vi "MD5 vs FileDateSize Check.vi"() -> ()   [LabVIEW 2016]
panel:
  out "x-y":u32
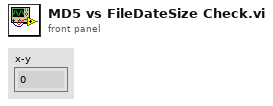
[diagram p1: front panel]
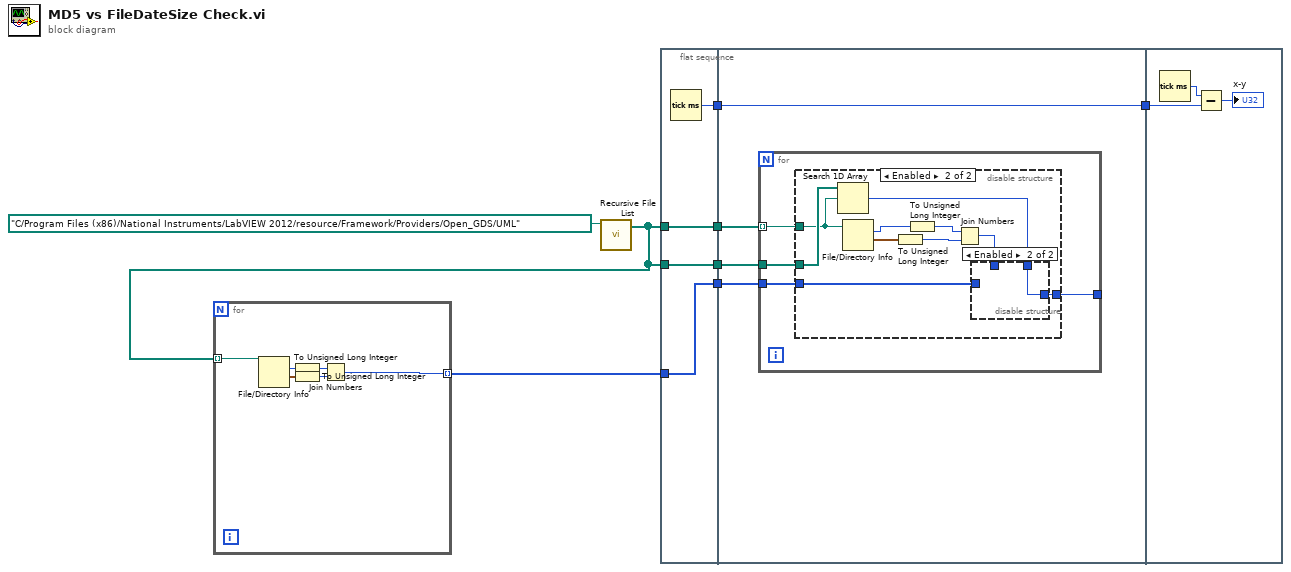
[diagram p0: block diagram]
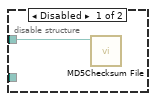
[diagram p2: hidden frame]
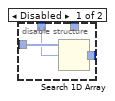
[diagram p3: hidden frame]
diagram:
  n1 = call <vilib>:"Recursive File List.vi"("Folder Path"=path "C:/Program Files (x86)/National Instruments/LabVIEW 2012/resource/Framework/Providers/Open_GDS/UML") -> ("All Files in Dir"=w2:path[])  [unwired: 6 in, 4 out]
  n2 = for {
    tunnel: w2 -> [w14] mode=indexing
    tunnel: [w13] -> w4 mode=indexing
    n3 = File/Directory Info(path=w14) -> (size=w11:i64, last mod=w12:timestamp)  [unwired: 1 in, 5 out]
    n4 = To Unsigned Long Integer(number=w11) -> (unsigned 32bit integer=w10:u32)
    n5 = To Unsigned Long Integer(number=w12) -> (unsigned 32bit integer=w9:u32)
    n6 = Join Numbers(hi=w10, lo=w9) -> ((hi.lo)=w13:u64)
  }
  n7 = flat-sequence {
    tunnel: [w18] -> w8
    tunnel: w2 -> [w17]
    tunnel: [w17] -> w5
    tunnel: w4 -> [w16]
    tunnel: [w16] -> w3
    tunnel: w2 -> [w15]
    tunnel: [w15] -> w1
    tunnel: w8 -> [w22]
    tunnel: [w22] -> w7
    tunnel: w5 -> [w21]
    tunnel: w3 -> [w20]
    tunnel: w1 -> [w19]
    tunnel: w7 -> [w43]
    frame #0 {
      n8 = Tick Count (ms)() -> (millisecond timer value=w18:u32)
    }
    frame #1 {
      n9 = for {
        tunnel: w21 -> [w26] mode=indexing
        tunnel: w20 -> [w25]
        tunnel: [w24] -> _
        tunnel: w19 -> [w23]
        n10 = disable-structure shown="Enabled" {
          disable-tunnel: w26 -> [w27 w29]
          disable-tunnel: w25 -> [_ w33]
          disable-tunnel: [_ w31] -> w24
          disable-tunnel: w23 -> [_ w30]
          frame Disabled {
            n11 = call <vilib>:"MD5Checksum File.vi"("Path"=w27) -> ()  [unwired: 9 in, 2 out]
          }
          frame Enabled {
            n12 = Search 1D Array(1D array=w30, element=w29) -> (index of element=w28:i32)  [unwired: 1 in]
            n13 = File/Directory Info(path=w29) -> (size=w35:i64, last mod=w34:timestamp)  [unwired: 1 in, 5 out]
            n14 = To Unsigned Long Integer(number=w34) -> (unsigned 32bit integer=w37:u32)
            n15 = To Unsigned Long Integer(number=w35) -> (unsigned 32bit integer=w36:u32)
            n16 = Join Numbers(hi=w36, lo=w37) -> ((hi.lo)=w32:u64)
            n17 = disable-structure shown="Enabled" {
              disable-tunnel: w33 -> [w40 _]
              disable-tunnel: w32 -> [w39 _]
              disable-tunnel: [w38 w41] -> w31
              disable-tunnel: w28 -> [_ w41]
              frame Disabled {
                n18 = Search 1D Array(1D array=w40, element=w39) -> (index of element=w38:i32)  [unwired: 1 in]
              }
              frame Enabled {
              }
            }
          }
        }
      }
    }
    frame #2 {
      n19 = Tick Count (ms)() -> (millisecond timer value=w44:u32)
      n20 = Subtract(x=w44, y=w43) -> (x-y=→"x-y":u32)
    }
  }
